vi "Test Create Logger with Rotating Daily File Sink as Default.vi"(11 "Test Case In":refnum<class "Rotating Daily File Sink.lvclass">) -> (0 "error out":errorcluster, 3 "Test Case Out":refnum<class "Rotating Daily File Sink.lvclass">)   [LabVIEW 2020, in "Rotating Daily File Sink.lvclass"]
uses:
  Rotating Daily File Sink.lvclass
  C:/Program Files (x86)/National Instruments/LabVIEW 2020/vi.lib/Astemes/LUnit/Test Case.lvclass
  Source/Type Defs/Debug Level.ctl
  <vilib>/Astemes/LUnit/Test Case.lvclass/Test Case.ctl
  e0c7a7cc-5830-4673-a67d-18354674fd35.vi
  89f79ace-e66e-4d1c-86d9-b8788306fe36.vi
  8a204fe8-34b0-47c8-92ee-980a1ea9d0a5.vi
  <vilib>/Astemes/LUnit/Core/LUnit Test Case/Private/Append Fail Result.vi
  <vilib>/Astemes/LUnit/Core/LUnit Test Case/Private/Append Pass Result.vi
  e0c7a7cc-5830-4673-a67d-18354674fd35.vi/9c5d11cd-9439-4240-a1ee-d9baace9c924.vi
  89f79ace-e66e-4d1c-86d9-b8788306fe36.vi/9c5d11cd-9439-4240-a1ee-d9baace9c924.vi
  8a204fe8-34b0-47c8-92ee-980a1ea9d0a5.vi/9c5d11cd-9439-4240-a1ee-d9baace9c924.vi
  <vilib>/Astemes/LUnit/Core/LUnit Test Case/Private/Run In UI.vi
  <vilib>/Utility/error.llb/Clear Errors.vi
  Source/Sinks/Rotating File Sink/Rotating Daily File Sink.lvclass
  C:/Users/hughe_cx/Documents/05_repos/LVLog/Source/Sinks/Sink/Sink.lvclass
  Rotating Daily File Sink.lvclass/Rotating Daily File Sink.ctl
  Source/LV Log.lvlib
  Source/Logger/Logger.lvclass
  <vilib>/Astemes/LUnit/Test Case.lvclass
  C:/Program Files (x86)/National Instruments/LabVIEW 2020/vi.lib/Astemes/LUnit/LUnit Runnable.lvclass
  C:/Users/hughe_cx/Documents/05_repos/LVLog/Testing/Rotating Daily File Sink/Rotating Daily File Sink.lvclass
  C:/Users/hughe_cx/Documents/05_repos/LVLog/Source/Sinks/File Sink/File Sink.lvclass
  C:/Users/hughe_cx/Documents/05_repos/LVLog/Source/Sinks/Rotating File Sink/Rotating Daily File Sink.lvclass
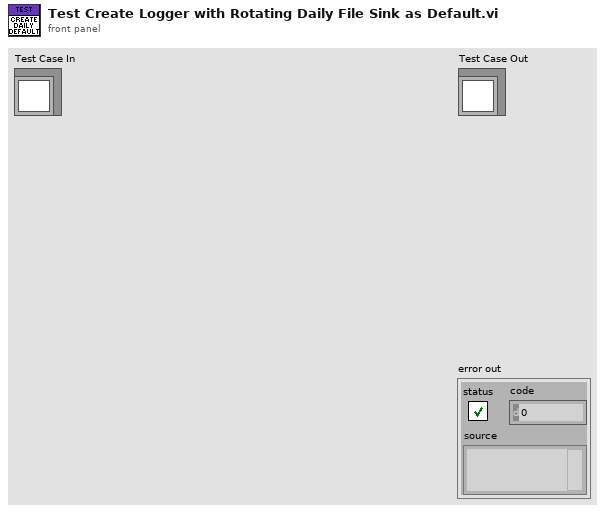
[diagram p1: front panel]
types:
  T1 = typedef "LV Log.lvlib/Debug Level.ctl" = enum16{"DEFAULT", "DEBUG", "INFO", "WARN", "ERROR", "FATAL"}
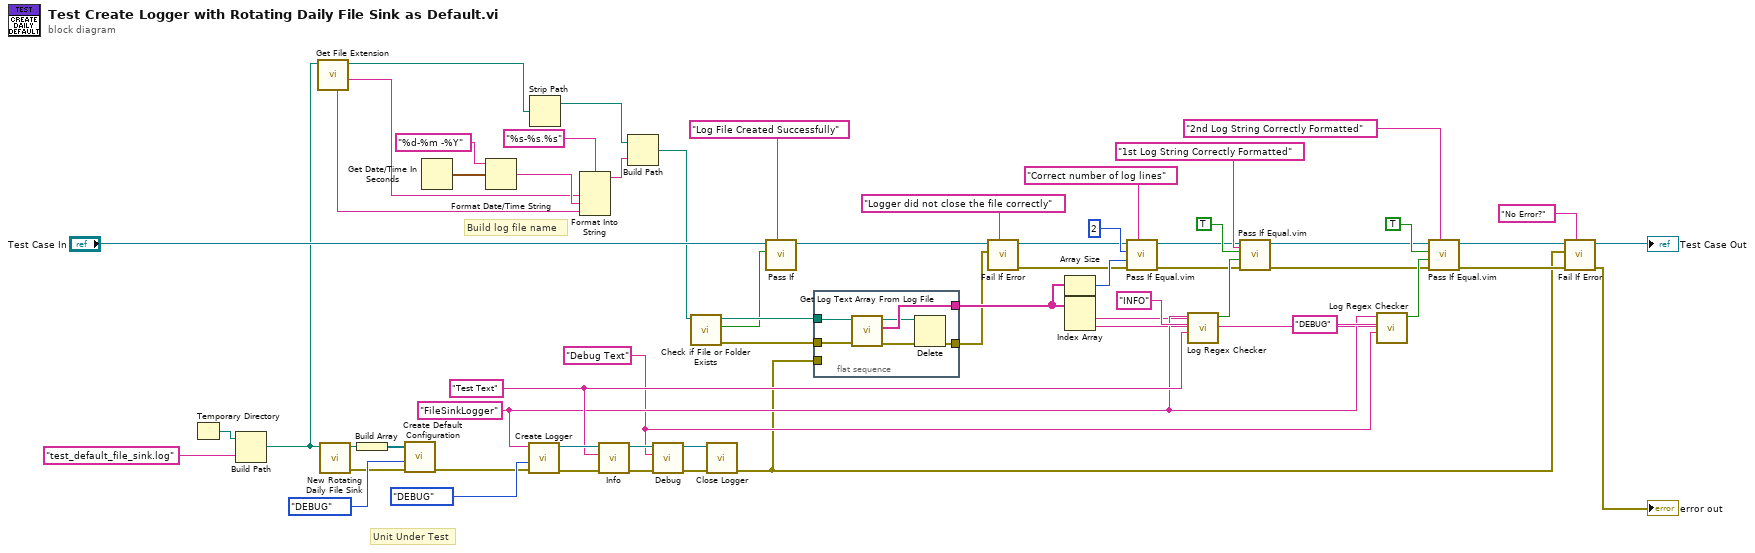
[diagram p0: block diagram]
diagram:
  w48 = "Debug Text" ("Log Text")
  w57 = "Test Text" ("Log Text")
  w49 = "FileSinkLogger" ("Name")
  # "Build log file name"
  # "Unit Under Test"
  n1 = Temporary Directory() -> (w62:path)
  n2 = Build Path(base path=w62, name or relative path="test_default_file_sink.log" ("format string")) -> (appended path=w7:path)
  n3 = call <vilib>:"Get File Extension.vi"("file"=w7) -> ("filename without extension"=w9:string, "dup file"=w5:path, "unmodified file extension"=w10:string)  [unwired: 6 in, 2 out]
  n4 = call "New Rotating Daily File Sink.vi"("File Path"=w7) -> ("error out"=w3:errorcluster, "Rotating Daily File Sink out"=w17:refnum<class "Rotating Daily File Sink.lvclass">)  [unwired: 9 in]
  n5 = Build Array(w17) -> (w2:refnum<class "Rotating Daily File Sink.lvclass">[])
  n6 = call "Create Default Configuration.vi"("Sinks"=w2, "Debug Level in"=Debug_Level."DEBUG", "error in (no error)"=w3) -> ("error out"=w1:errorcluster)  [unwired: 7 in]
  n7 = Get Date/Time In Seconds() -> (seconds since 1Jan1904=w13:timestamp)
  n8 = Format Date/Time String(time format string (%c)="%d-%m -%Y", seconds (now)=w13) -> (date/time string=w14:string)  [unwired: 1 in]
  n9 = call "Create Logger.vi"("error in (no error)"=w1, "Debug Level (Default)"=Debug_Level."DEBUG" ("Debug Level in"), "Name"=w49) -> ("error out"=w61:errorcluster, "Logger out"=w60:refnum<class "Logger.lvclass">)  [unwired: 7 in]
  n10 = Strip Path(path=w5) -> (stripped path=w11:path)  [unwired: 1 out]
  n11 = Format Into String(format string="%s-%s.%s", w9, w14, w10) -> (resulting string=w12:string)  [unwired: 2 in, 1 out]
  n12 = call "Info.vi"("error in (no error)"=w61, "Log Text"=w57, "Logger in"=w60) -> ("error out"=w56:errorcluster, "Logger out"=w55:refnum<class "Logger.lvclass">)  [unwired: 6 in, 1 out]
  n13 = Build Path(base path=w11, name or relative path=w12) -> (appended path=w6:path)
  n14 = call "Debug.vi"("error in (no error)"=w56, "Log Text"=w48, "Logger in"=w55) -> ("error out"=w31:errorcluster, "Logger out"=w30:refnum<class "Logger.lvclass">)  [unwired: 6 in, 1 out]
  n15 = call <vilib>:"Check if File or Folder Exists.vi"("path"=w6) -> ("error out"=w35:errorcluster, "file or folder exists?"=w34:bool, "dup path"=w36:path)  [unwired: 8 in]
  n16 = call "Close Logger.vi"("error in (no error)"=w31, "Logger in"=w30) -> ("error out"=w29:errorcluster)  [unwired: 9 in]
  n17 = call <vilib>:"Pass If.vi"("Description"="Log File Created Successfully", "Pass?"=w34, "LUnit Test Case In"="Test Case In") -> ("LUnit Test Case Out"=w26:refnum<class "Rotating Daily File Sink.lvclass">)  [unwired: 7 in, 1 out]
  n18 = flat-sequence {
    tunnel: w36 -> [w68]
    tunnel: [w67] -> w42
    tunnel: w35 -> [w64]
    tunnel: w29 -> [_]
    tunnel: [w63] -> w22
    frame #0 {
      n19 = call "Get Log Text Array From Log File.vi"("error in"=w64, "Log File Path in"=w68) -> ("error out"=w66:errorcluster, "Log Text Array"=w67:string[], "Log File Path out"=w65:path)  [unwired: 7 in]
      n20 = Delete(path (use dialog)=w65, error in=w66) -> (error out=w63:errorcluster)  [unwired: 3 in, 2 out]
    }
  }
  n21 = call <vilib>:"Fail If Error.vi"("Description"="Logger did not close the file correctly", "Assert error"=w22, "LUnit Test Case In"=w26) -> ("error out"=w23:errorcluster, "LUnit Test Case Out"=w25:refnum<class "Rotating Daily File Sink.lvclass">)  [unwired: 7 in]
  n22 = Array Size(array=w42) -> (size(s)=w41:i32)
  n23 = Index Array(array=w42) -> (element #1=w47:string, element #2=w46:string)  [unwired: 2 in]
  n24 = call "Pass If Equal.vim"("Description"="Correct number of log lines", "error in (no error)"=w23, "Actual"=w41, "Expected"=2, "LUnit Test Case In"=w25) -> ("error out"=w37:errorcluster, "LUnit Test Case Out"=w43:refnum<class "Rotating Daily File Sink.lvclass">)  [unwired: 5 in]
  n25 = call "Log Regex Checker.vi"("Log String"=w47, "Expected Log Text (Any)"=w57, "Expected Log Level (Any)"="INFO", "Expected Logger Name (Any)"=w49) -> ("Math Found"=w53:bool)  [unwired: 5 in, 2 out]
  n26 = call "Pass If Equal.vim"("Description"="1st Log String Correctly Formatted", "error in (no error)"=w37, "Actual"=w53, "Expected"=TRUE, "LUnit Test Case In"=w43) -> ("error out"=w38:errorcluster, "LUnit Test Case Out"=w45:refnum<class "Rotating Daily File Sink.lvclass">)  [unwired: 5 in]
  n27 = call "Log Regex Checker.vi"("Log String"=w46, "Expected Log Text (Any)"=w48, "Expected Log Level (Any)"="DEBUG", "Expected Logger Name (Any)"=w49) -> ("Math Found"=w52:bool)  [unwired: 5 in, 2 out]
  n28 = call "Pass If Equal.vim"("Description"="2nd Log String Correctly Formatted", "error in (no error)"=w38, "Actual"=w52, "Expected"=TRUE, "LUnit Test Case In"=w45) -> ("error out"=w39:errorcluster, "LUnit Test Case Out"=w44:refnum<class "Rotating Daily File Sink.lvclass">)  [unwired: 5 in]
  n29 = call <vilib>:"Fail If Error.vi"("Description"="No Error?", "error in (no error)"=w39, "Assert error"=w29, "LUnit Test Case In"=w44) -> ("error out"=→"error out":errorcluster, "LUnit Test Case Out"=→"Test Case Out":refnum<class "Rotating Daily File Sink.lvclass">)  [unwired: 6 in]
